vi "Panel - Calibration.vi"() -> ()   [LabVIEW 2020]
doc: "Panel to hold all calibration controls"
uses:
  Library - Test Executive.llb/Test Executive - Globals.vi
panel:
  in  "stop":bool
  in  "Check Test Equipment":bool
  out "errors":errorcluster
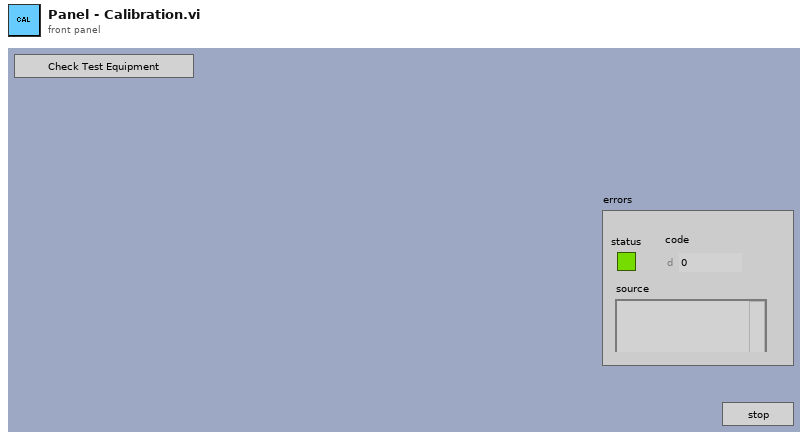
[diagram p1: front panel]
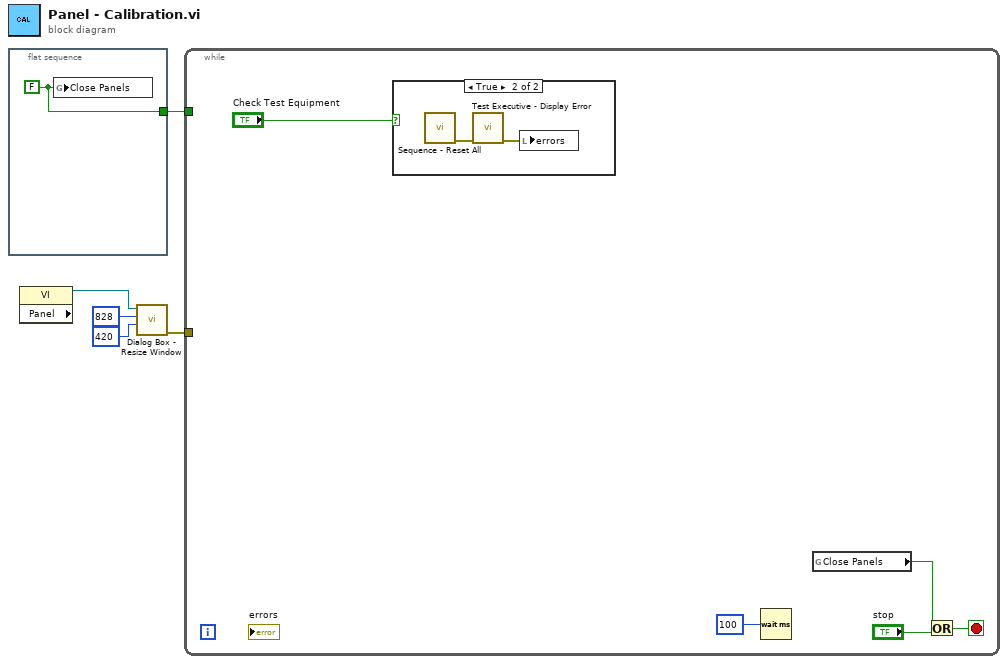
[diagram p0: block diagram]
diagram:
  n1 = flat-sequence {
    tunnel: [w6] -> w5
    frame #0 {
      w6 = FALSE ("Close Panels")
      n2 = global write "Test Executive - Globals.vi" "Close Panels"(w6) -> ()
    }
  }
  n3 = property class="VI" props=["Panel"]() -> (reference out=w2:refnum<vi>)  [unwired: 2 in, 2 out]
  n4 = call "Dialog Box - Resize Window.vi"("Height"=i16 420, "Width"=i16 828, "reference"=w2) -> ("error out"=w1:errorcluster)  [unwired: 8 in]
  n5 = while {
    tunnel: w5 -> [_]
    tunnel: w1 -> [_]
    stop <- w8 stop-if-true
    n6 = case shown="True" "Check Test Equipment" {
      frame False {
      }
      frame True {
        n7 = call "Sequence - Reset All.vi"() -> ("error out"=w13:errorcluster)  [unwired: 11 in]
        n8 = call "Test Executive - Display Error.vi"("error in (no error)"=w13) -> ("error out"=w12:errorcluster)  [unwired: 10 in]
        n9 = local write "errors"(w12) -> ()
      }
    }
    n10 = Wait (ms)(milliseconds to wait=u32 100) -> ()  [unwired: 1 out]
    n11 = global read "Test Executive - Globals.vi" "Close Panels"() -> (w9:bool)
    n12 = Or(x=w9, y="stop") -> (x .or. y?=w8:bool)
  }
